vi "fill-dense-template_v1.0.vi"() -> ()   [LabVIEW 2020]
uses:
  <vilib>/Analysis/7linalg.llb/Real Transpose Matrix.vi
  <vilib>/Analysis/Matrix/Numeric/Conversions/Array To Matrix - RA2.vi
  <vilib>/Analysis/Matrix/Numeric/Conversions/Matrix To Array - RM.vi
  <vilib>/Analysis/NI_AALPro.lvlib
  <vilib>/Analysis/Matrix/NI_Matrix.lvlib
panel:
  in  "weight path":path
  in  "name":string
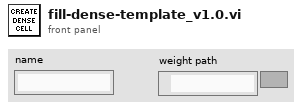
[diagram p1: front panel]
types:
  T1 = typedef "NI_Matrix.lvlib/RealMatrix.ctl" = dbl[][]
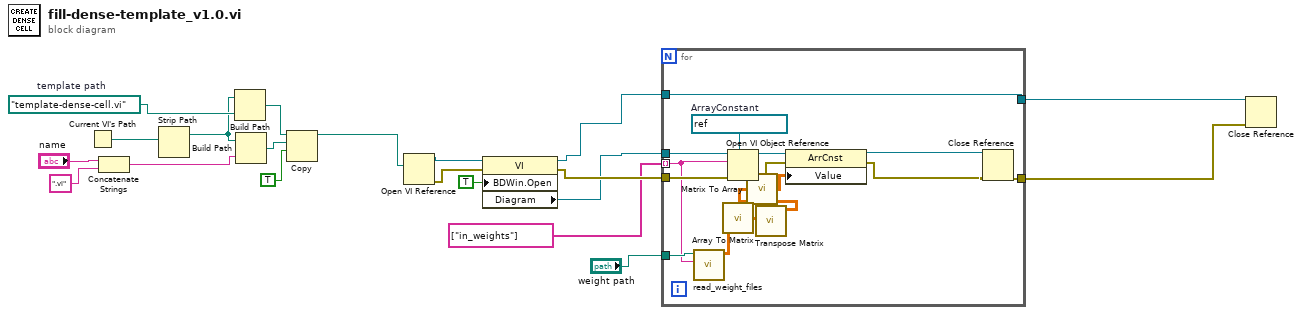
[diagram p0: block diagram]
diagram:
  w4 = path "template-dense-cell.vi"  # template path
  n1 = Current VI's Path() -> (path=w2:path)
  n2 = Concatenate Strings("name", ".vi") -> (w13:string)
  n3 = Strip Path(path=w2) -> (stripped path=w1:path)  [unwired: 1 out]
  n4 = Build Path(base path=w1, name or relative path=w4) -> (appended path=w3:path)
  n5 = Build Path(base path=w1, name or relative path=w13) -> (appended path=w12:path)
  n6 = Copy(9:TRUE, 10:w12, 11:w3) -> (3:w8:path)  [unwired: 2 in, 2 out]
  n7 = Open VI Reference(vi path=w8) -> (vi reference=w10:refnum<vi>, error out=w9:errorcluster)  [unwired: 5 in]
  n8 = property class="VI"(reference=w10, error in=w9, "BDWin.Open"=TRUE) -> (reference out=w6:refnum<vi>, error out=w17:errorcluster, "Diagram"=w7:refnum<vi>)
  n9 = for {
    tunnel: w17 -> [w35]
    tunnel: w7 -> [w34]
    tunnel: string[] ["in_weights"] -> [w25] mode=indexing
    tunnel: [w29] -> w20
    tunnel: "weight path" -> [w26]
    tunnel: [w30] -> w16
    tunnel: w6 -> [w30]
    w33 = refnum<vi> refnum  # ArrayConstant
    n10 = call "read_weight_files.vi"("weight file name"=w25, "weights path"=w26) -> ("all rows"=w24:dbl[][])  [unwired: 9 in]
    n11 = call-poly <vilib>:"Array To Matrix.vi"("Real 2D Array"=w24) -> ("Real Matrix"=w23:T1)
    n12 = Open VI Object Reference(7:w33, 8:w35, 10:w25, 11:w34) -> (0:w31:errorcluster, 3:w32:refnum<vi>)
    n13 = call-poly <vilib>:"Transpose Matrix.vi"("Input Matrix"=w23) -> ("Matrix Transpose"=w22:T1)  [unwired: 9 in, 1 out]
    n14 = call-poly <vilib>:"Matrix To Array.vi"("Real Matrix"=w22) -> ("Real 2D Array"=w21:dbl[][])
    n15 = property class="ArrCnst"(reference=w32, error in=w31, "Value"=w21) -> (reference out=w28:refnum<vi>, error out=w27:errorcluster)
    n16 = Close Reference(reference=w28, error in (no error)=w27) -> (error out=w29:errorcluster)
  }
  n17 = Close Reference(reference=w16, error in (no error)=w20) -> ()  [unwired: 1 out]
